vi "Read Sys Log.vi"(8 "error in (no error)":errorcluster, 11 "Serial Session in":refnum<class "Serial Session.lvclass">) -> (0 "error out":errorcluster, 2 "Session Handle":T1, 3 "Serial Session out":refnum<class "Serial Session.lvclass">)   [LabVIEW 2015, in "Serial Session.lvclass"]
uses:
  Serial Session.lvclass
  _Session Fwk/Typedefs/Session Handle.ctl
  _Session Fwk/Session - Root.lvclass
  Serial Session.lvclass/Serial Session.ctl
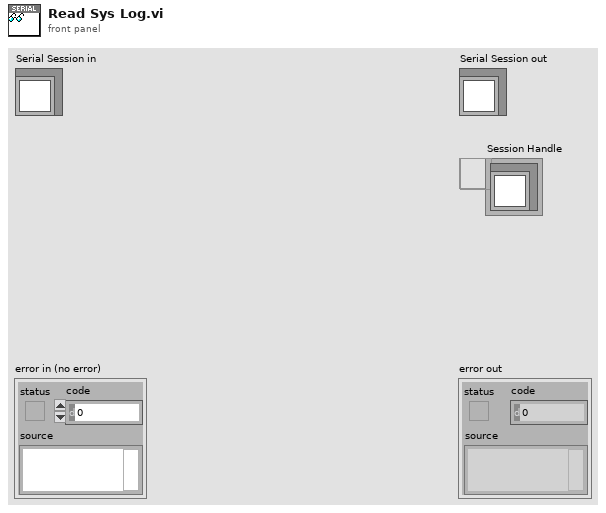
[diagram p1: front panel]
types:
  T1 = typedef "Session - Root.lvclass/Session Handle.ctl" = refnum<data-value>
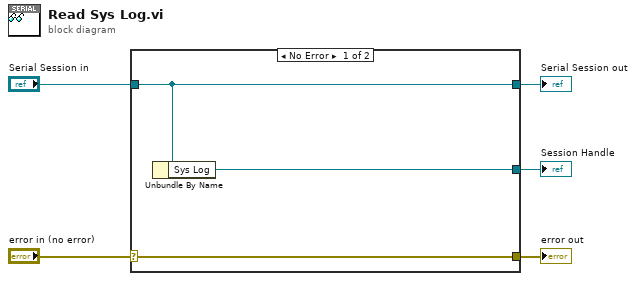
[diagram p0: block diagram]
diagram:
  n1 = case shown="No Error" "error in (no error)" {
    selector: "error in (no error)" -> [w8 w9]
    tunnel: [w8 w9] -> w4
    tunnel: [w7 w10] -> w2
    tunnel: "Serial Session in" -> [w7 w10]
    tunnel: [w6 _] -> w1
    frame No Error {
      n2 = Unbundle By Name(w7) -> ("Sys Log"=w6:T1)
    }
    frame Error {
    }
  }
  "error out" <- w4
  "Serial Session out" <- w2
  "Session Handle" <- w1
